vi "g4_type.vi"(11 "Line in":string) -> (1 "Line out":string, 3 "G4 type":T1=enum."G4 previous line pause")   [LabVIEW 2017, in "labview-standard-library.lvlib" / "automode-scripting.lvlib"]
uses:
  automode-scripting.lvlib
  type-defs/execution_stop_type.ctl
  <vilib>/regexp/Match Regular Expression.xnode
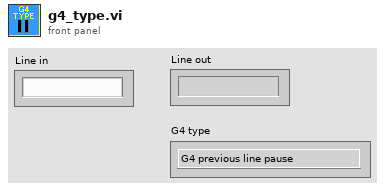
[diagram p1: front panel]
types:
  T1 = typedef "labview-standard-library.lvlib/automode-scripting.lvlib/execution_stop_type.ctl" = enum16{"G4 timed pause", "G4 previous line pause", "G4 tool pause", "M0 Breakpoint", "Invalid"}
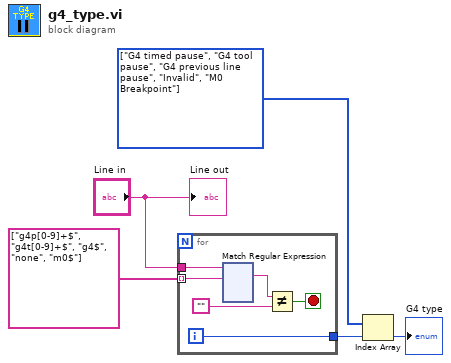
[diagram p0: block diagram]
diagram:
  w3 = T1[] [enum."G4 timed pause", enum."G4 tool pause", enum."G4 previous line pause", enum."Invalid", enum."M0 Breakpoint"] items=["G4 timed pause", "G4 previous line pause", "G4 tool pause", "M0 Breakpoint", "Invalid"]
  n1 = for {
    tunnel: "Line in" -> [w9]
    tunnel: string[] ["g4p[0-9]+$", "g4t[0-9]+$", "g4$", "none", "m0$"] -> [w8] mode=indexing
    tunnel: [w10] -> w2
    i -> [w10]
    stop <- w11 stop-if-true
    n2 = xnode "Match Regular Expression"("input string"=w9, "regular expression"=w8) -> ("whole match"=w7:string)  [unwired: 4 in, 4 out]
    n3 = Not Equal?(x=w7, y="") -> (x != y?=w11:bool)
  }
  n4 = Index Array(array=w3, index=w2) -> (element=→"G4 type":T1)
  "Line out" <- "Line in"
